vi "Init(Config) Global Log.vi"(8 "error in (no error)":errorcluster, 9 "iName":string, 10 "iType":string, 11 "Global Application Log in":refnum<class "Global Application Log.lvclass">) -> (0 "error out":errorcluster, 3 "Global Application Log out":refnum<class "Global Application Log.lvclass">)   [LabVIEW 2016, in "Stream Log.lvlib" / "Global Application Log.lvclass"]
doc: "--\nCopyright © 2017 Composed SystemsI All rights reserved.\n\nAuthor: Jon McBee <jon.mcbee@composed.io>\n\nThis library is provided \"AS IS\" ,WITHOUT WARRANTIES OR\nCONDITIONS OF ANY KIND, either express or implied.\n\nComposed Systems -- composed.io\n\nStream 0.0.1.1\nJon McBee - Composed Systems\nCopyright (c) 2017, Composed Systems"
uses:
  <userlib>/Composed Systems/Stream/Log/Global Application Log/Global Application Log.lvclass
  C:/Program Files (x86)/National Instruments/LabVIEW 2016/user.lib/Composed Systems/Stream/Actor/Actor Class/Ancestral Actor.lvclass
  <userlib>/Composed Systems/Stream/Actor/Actor Class/Ancestral Actor.lvclass/Ancestral Actor.ctl
  <userlib>/Composed Systems/Stream/Actor/Actor Class/Ancestral Actor.lvclass
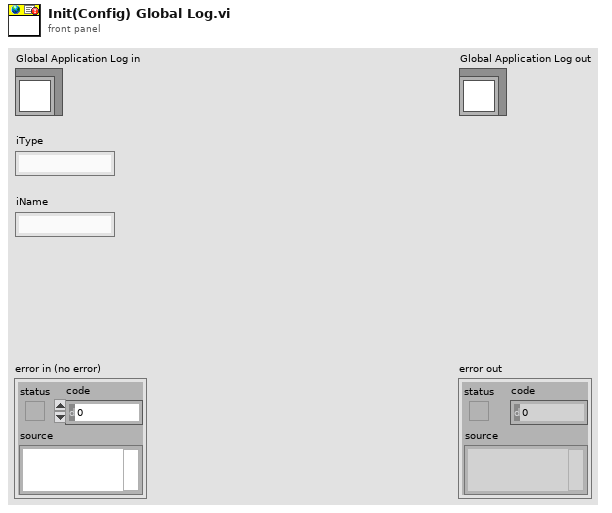
[diagram p1: front panel]
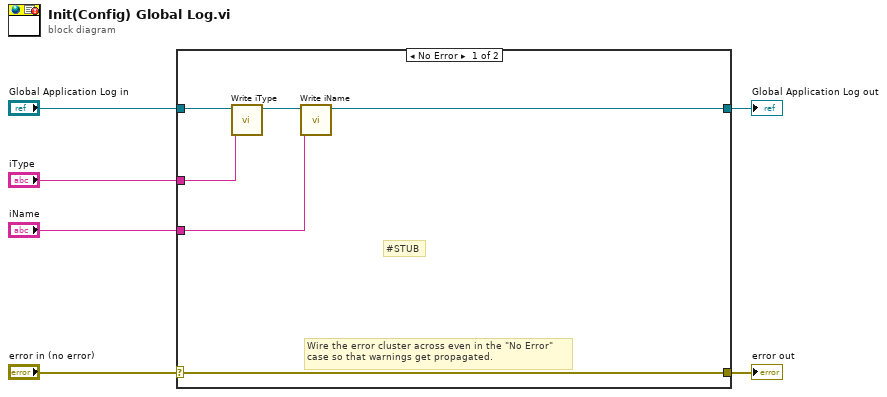
[diagram p0: block diagram]
diagram:
  n1 = case shown="No Error" "error in (no error)" {
    selector: "error in (no error)" -> [w12 w14]
    tunnel: [w12 w14] -> w5
    tunnel: [w9 w13] -> w3
    tunnel: "Global Application Log in" -> [w10 w13]
    tunnel: "iType" -> [w8 _]
    tunnel: "iName" -> [w7 _]
    frame No Error {
      # "#STUB"
      # "Wire the error cluster across even in the \"No Error\"\ncase so that warnings get propagated."
      n2 = call <userlib>:"Write iType.vi"("iType"=w8, "Ancestral Actor in"=w10) -> ("Ancestral Actor out"=w11:refnum<class "Global Application Log.lvclass">)  [unwired: 8 in, 1 out]
      n3 = call <userlib>:"Write iName.vi"("iName"=w7, "Ancestral Actor in"=w11) -> ("Ancestral Actor out"=w9:refnum<class "Global Application Log.lvclass">)  [unwired: 8 in, 1 out]
    }
    frame Error {
    }
  }
  "error out" <- w5
  "Global Application Log out" <- w3
